vi "muestrapokemon.vi"() -> ()   [LabVIEW 2016]
panel:
  out "new picture":picture
  out "filenames":string[](array[string])
  in  "File Path Control":path
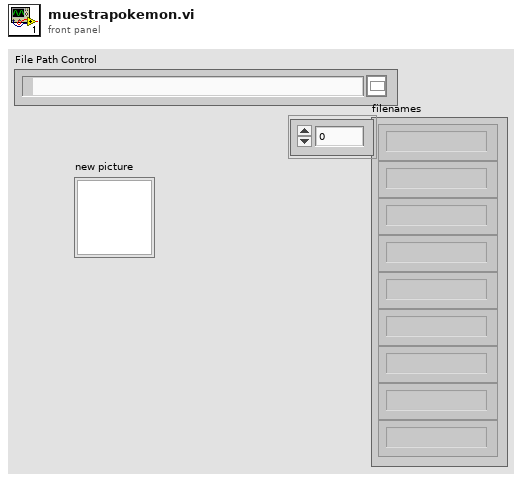
[diagram p1: front panel]
types:
  T1 = typedef "imagedata.ctl" = cluster{"image type":i32, "image depth":i32, "image":u8[], "mask":u8[], "colors":u32[], "Rectangle":cluster{"left":i16, "top":i16, "right":i16, "bottom":i16}}
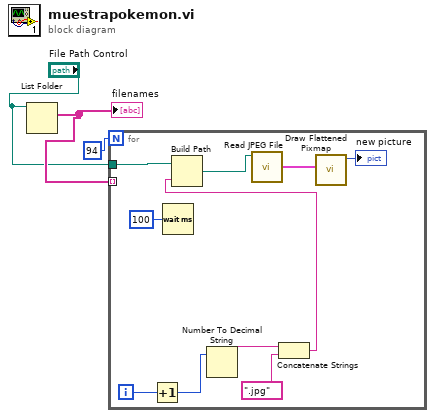
[diagram p0: block diagram]
diagram:
  n1 = List Folder(path="File Path Control") -> (filenames=w3:string[])  [unwired: 3 in, 3 out]
  "filenames" <- w3
  n2 = for {
    N: 94 -> [_]
    tunnel: w3 -> [_] mode=indexing
    tunnel: "File Path Control" -> [w13]
    i -> [w8]
    n3 = Increment(x=w8) -> (x+1=w7:i32)
    n4 = Wait (ms)(milliseconds to wait=u32 100) -> ()  [unwired: 1 out]
    n5 = Number To Decimal String(number=w7) -> (decimal integer string=w6:string)  [unwired: 1 in]
    n6 = Concatenate Strings(w6, ".jpg" ("string")) -> (w4:string)
    n7 = Build Path(base path=w13, name or relative path=w4) -> (appended path=w11:path)
    n8 = call <vilib>:"Read JPEG File.vi"("path to JPEG file"=w11) -> ("image data"=w12:T1)  [unwired: 8 in, 2 out]
    n9 = call <vilib>:"Draw Flattened Pixmap.vi"("image data"=w12) -> ("new picture"=→"new picture":picture)  [unwired: 8 in]
  }
